vi "Course project.vi"() -> ()   [LabVIEW 2013]
uses:
  Controls/Car Race Cmd Data Cluster.ctl
  Controls/Car Race States.ctl
  Controls/Log Data Staus.ctl
  Controls/Car race Msg.ctl
  <vilib>/Utility/inputDevices.llb/keyboardAcquire.vi
panel:
  out "Speed":string
  in  "Re-Start":bool=TRUE
  out "Game Over":string
  out "Bonus":string
  out "New High Score":string
  out "Car Yellow":bool
  out "Car Race Indicator":T1
  out "User Profile":u16(ring)
  out "Message":string
  in  "Start":bool
  in  "Sign In":T2
  in  "Stop":bool
  out "Car Red":bool
  out "Race Track":u16(ring)
  # "User ID-"
  # "Password-"
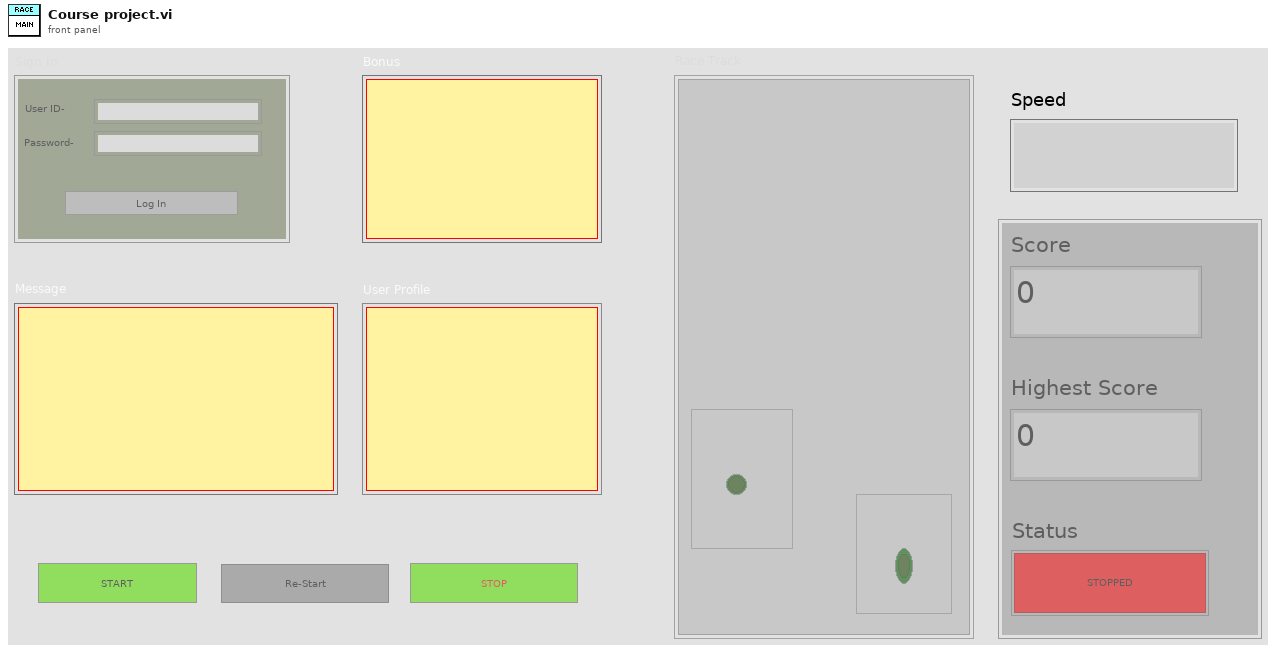
[diagram p1: front panel]
types:
  T1 = cluster{"Score":dbl, "Highest Score":dbl, "Status":bool}
  T2 = cluster{"User ID":string, "Password":string, "Log In":bool}
  T3 = typedef "Car Race Cmd Data Cluster.ctl" = cluster{"Command":T4, "Data":variant}
  T4 = typedef "Car Race States.ctl" = enum16{"Initialize", "Sign In", "Start", "Re-Start", "Game Over", "Stop"}
  T5 = cluster{"Sign In":refnum<vi>, "Race Track":refnum<vi>, "Car Red":refnum<vi>, "Car Yellow":refnum<vi>, "Car Race Indicator":refnum<vi>, "Start":refnum<vi>, "Stop":refnum<vi>, "Speed":refnum<vi>, "Re-Start":refnum<vi>}
  T6 = typedef "Car race Msg.ctl" = enum16{"Welcome Messsage", "User Inf.", "Start", "Log In Failed", "Game Over"}
  T7 = enum8{"Enabled", "Disabled", "Disabled and Grayed Out"}
  T8 = typedef "Log Data Staus.ctl" = enum16{"Initialize", "Read", "User ID Check", "Write", "Stop"}
  T9 = cluster{"First Name":string, "Last Name":string, "User ID":string, "Password":string, "Highest Score":string}
  T10 = cluster{"First Name":string, "Last Name":string, "User ID":string, "Password":string, "Highest Score":string}[]
  T11 = enum16{"0", "1", "2", "3", "4", "5", "6", "7", "8", "9", "A", "B", "C", "D", "E", "F", "G", "H", "I", "J", "K", "L", "M", "N", "O", "P", "Q", "R", "S", "T", "U", "V", "W", "X", "Y", "Z", "F1", "F2", "F3", "F4", "F5", "F6", "F7", "F8", "F9", "F10", "F11", "F12", "F13", "F14", "F15", "ADD", "BACK", "BACKSLASH", "CAPITAL", "COMMA", "DECIMAL", "DELETE", "DIVIDE", "DOWN", "END", "EQUALS", "ESCAPE", "GRAVE (`)", "HOME", "INSERT", "LBRACKET", "LCONTROL", "LEFT", "L ALT", "LSHIFT", "LWIN", "MINUS", "MULTIPLY", "NEXT", "NUMLOCK", "NUMPAD_0", "NUMPAD_1", "NUMPAD_2", "NUMPAD_3", "NUMPAD_4", "NUMPAD_5", "NUMPAD_6", "NUMPAD_7", "NUMPAD_8", "NUMPAD_9", "PAUSE", "PERIOD", "PRIOR (PG UP)", "RBRACKET", "RCONTROL", "RETURN", "RIGHT", "R ALT", "RSHIFT", "RWIN", "SCROLL", "SEMICOLON", "SLASH", "SPACE", "SUBTRACT", "TAB", "UP", "ENTER (num pad)", "' (quote)"}[]
  T12 = enum16{"0", "1", "2", "3", "4", "5", "6", "7", "8", "9", "A", "B", "C", "D", "E", "F", "G", "H", "I", "J", "K", "L", "M", "N", "O", "P", "Q", "R", "S", "T", "U", "V", "W", "X", "Y", "Z", "F1", "F2", "F3", "F4", "F5", "F6", "F7", "F8", "F9", "F10", "F11", "F12", "F13", "F14", "F15", "ADD", "BACK", "BACKSLASH", "CAPITAL", "COMMA", "DECIMAL", "DELETE", "DIVIDE", "DOWN", "END", "EQUALS", "ESCAPE", "GRAVE (`)", "HOME", "INSERT", "LBRACKET", "LCONTROL", "LEFT", "L ALT", "LSHIFT", "LWIN", "MINUS", "MULTIPLY", "NEXT", "NUMLOCK", "NUMPAD_0", "NUMPAD_1", "NUMPAD_2", "NUMPAD_3", "NUMPAD_4", "NUMPAD_5", "NUMPAD_6", "NUMPAD_7", "NUMPAD_8", "NUMPAD_9", "PAUSE", "PERIOD", "PRIOR (PG UP)", "RBRACKET", "RCONTROL", "RETURN", "RIGHT", "R ALT", "RSHIFT", "RWIN", "SCROLL", "SEMICOLON", "SLASH", "SPACE", "SUBTRACT", "TAB", "UP", "ENTER (num pad)", "' (quote)"}
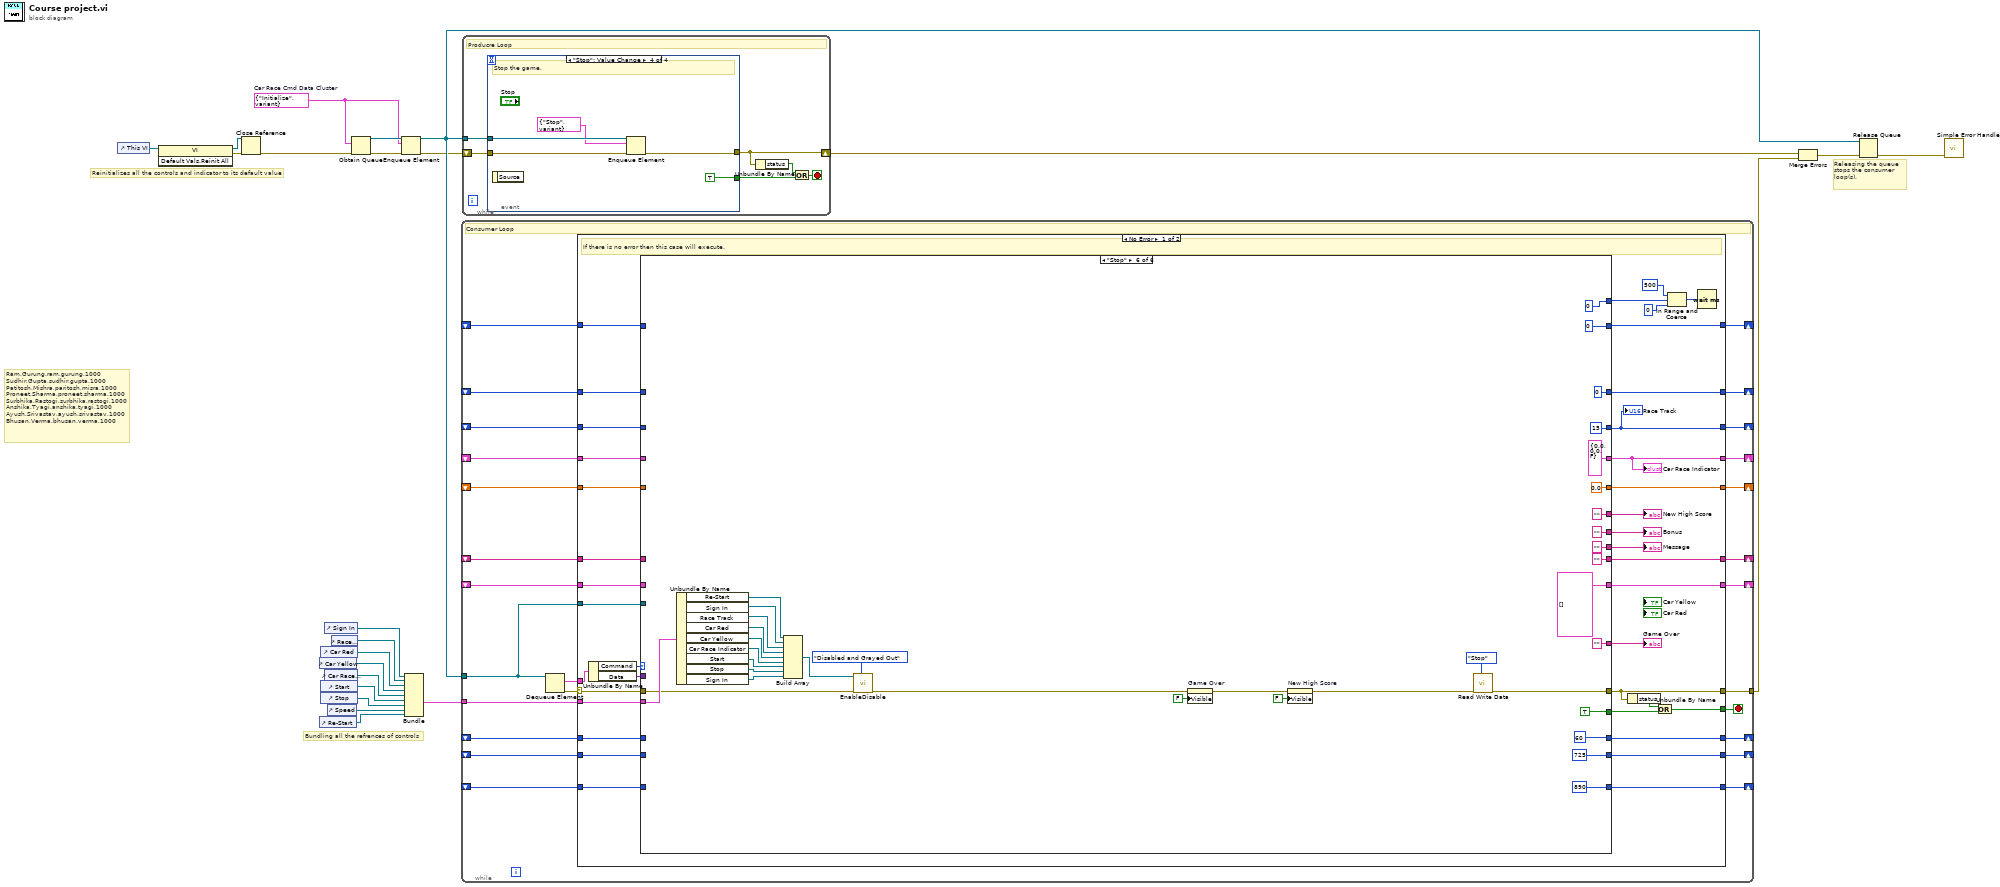
[diagram p0: block diagram]
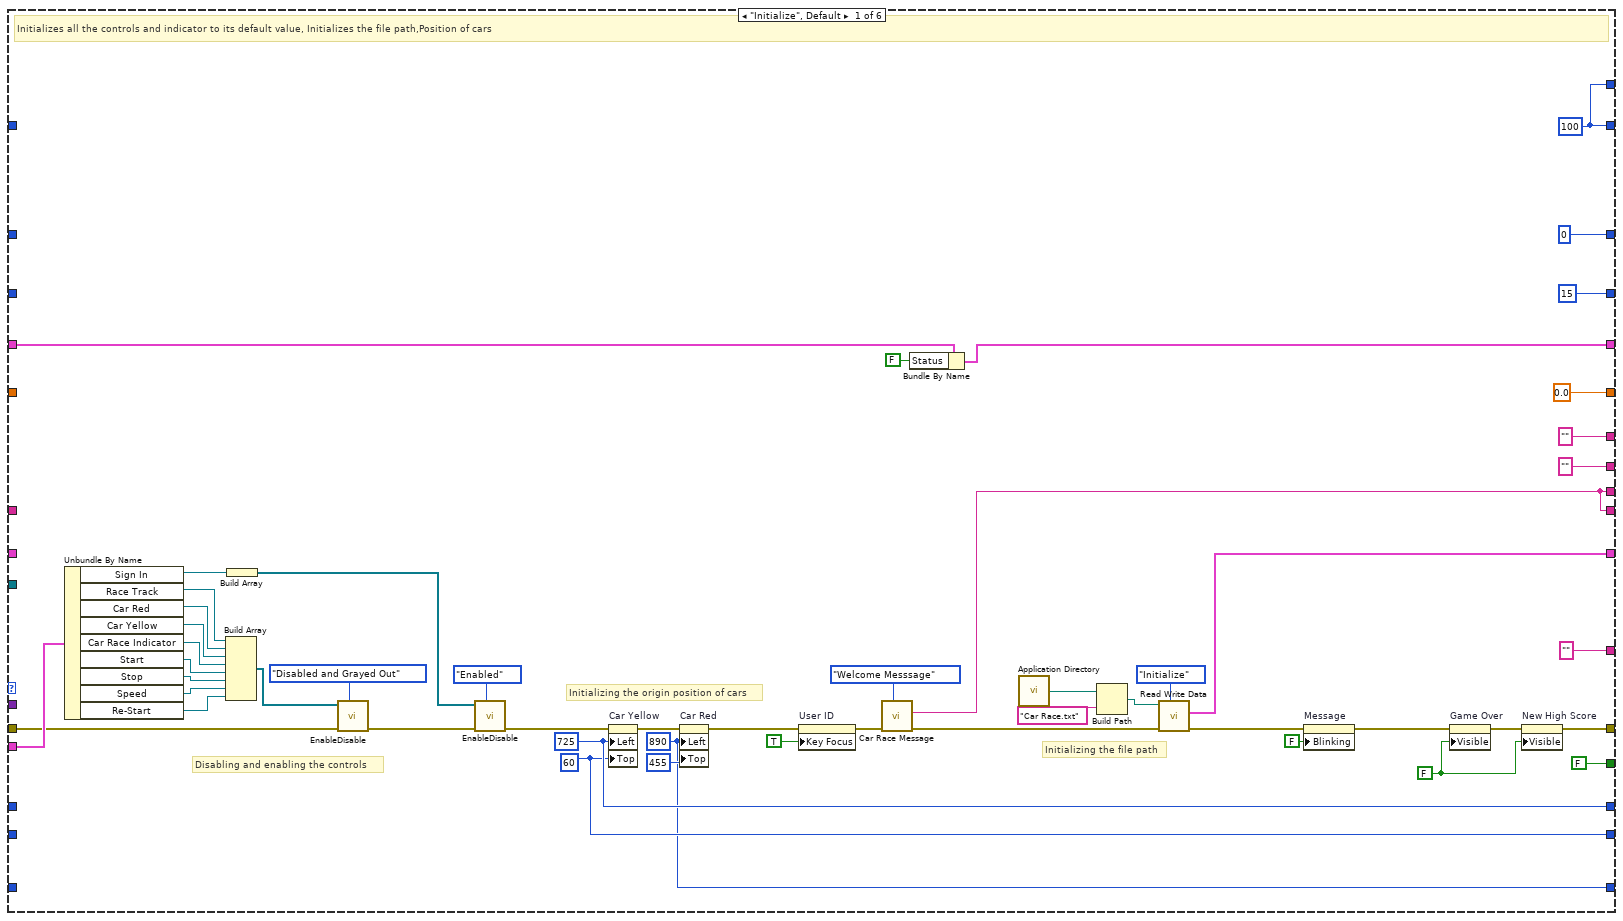
[diagram p2: hidden frame]
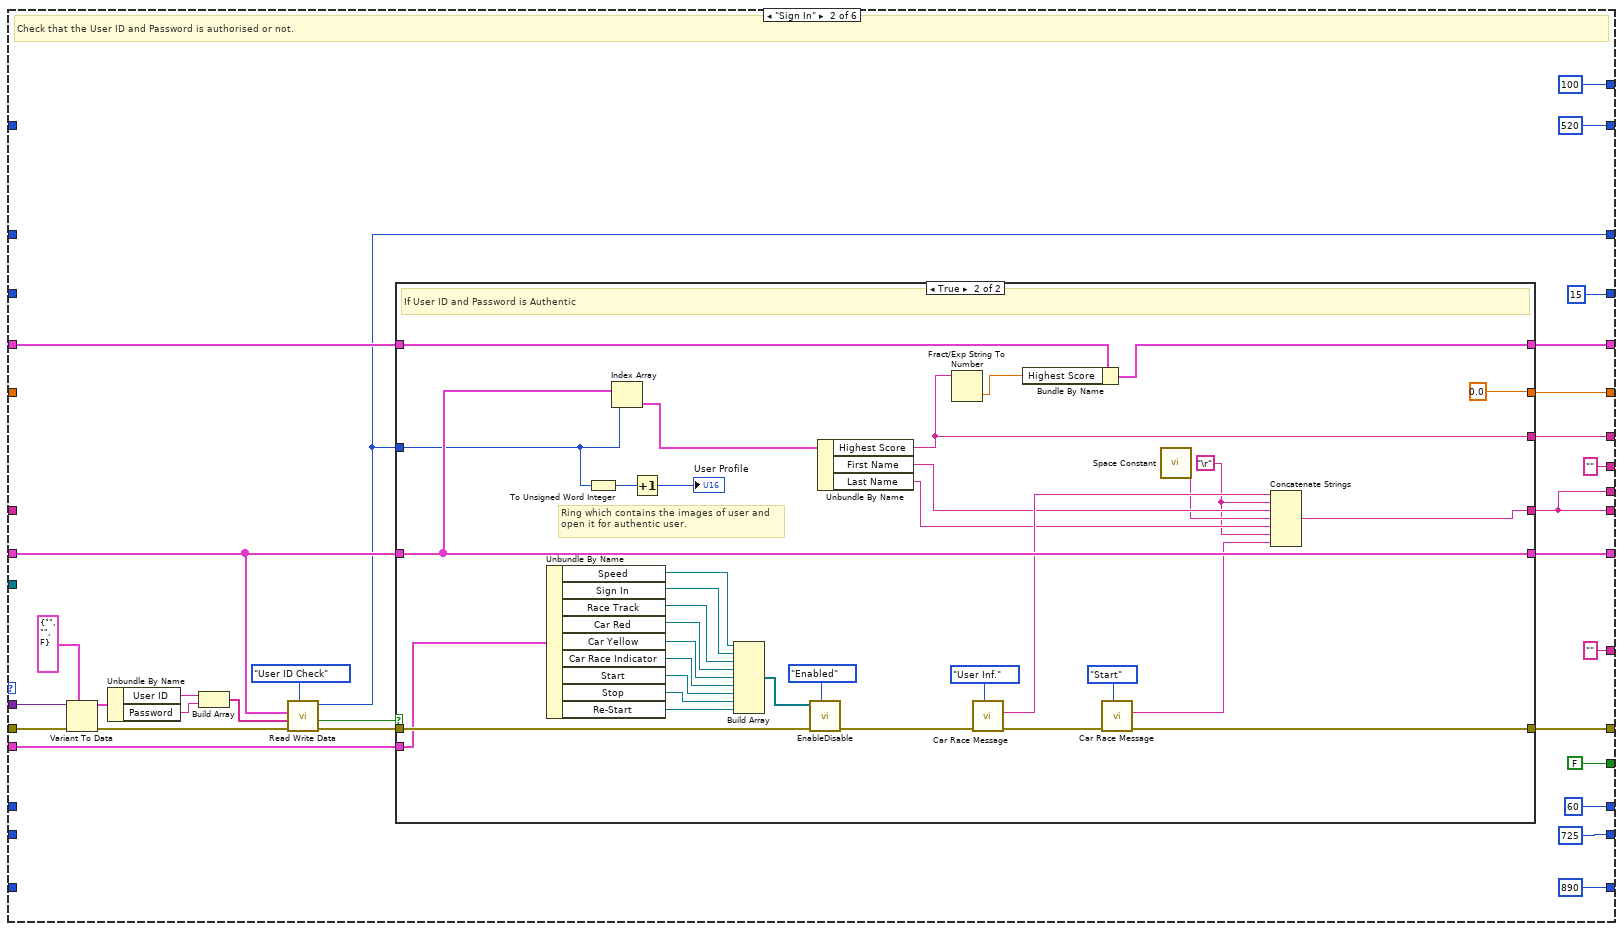
[diagram p3: hidden frame]
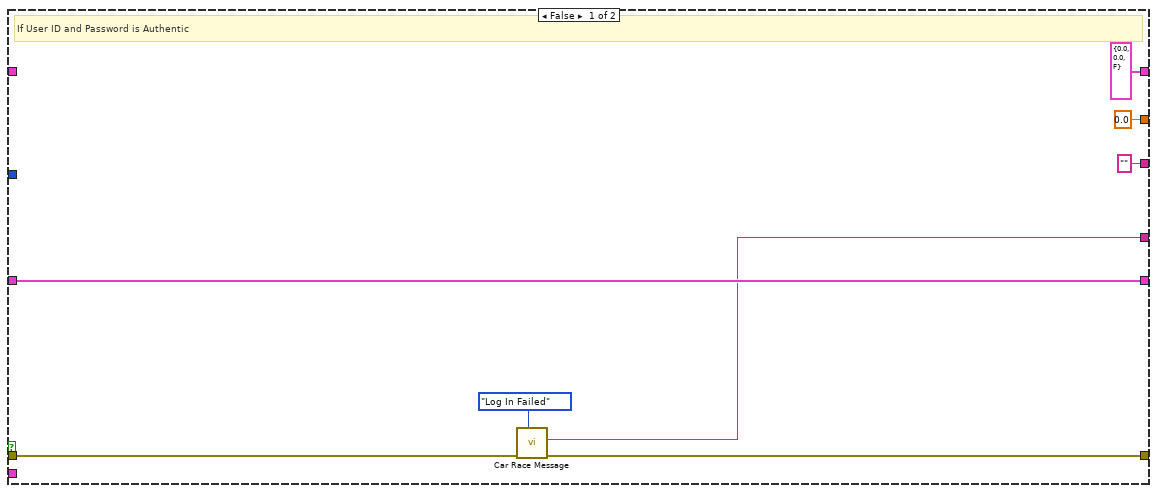
[diagram p4: hidden frame]
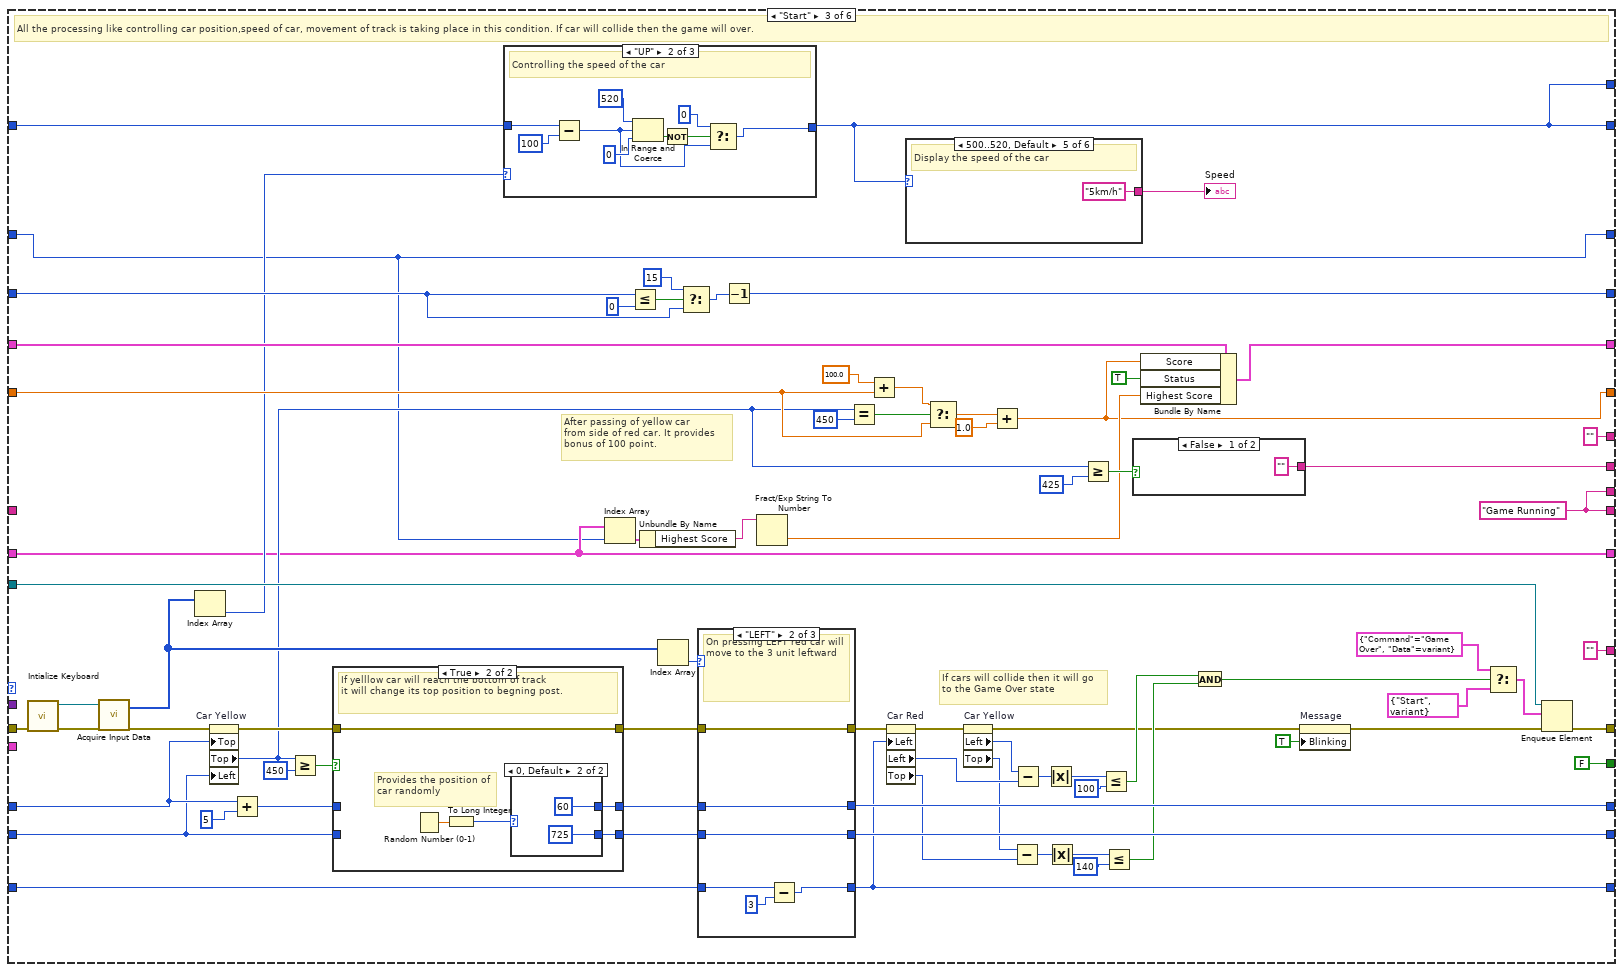
[diagram p5: hidden frame]
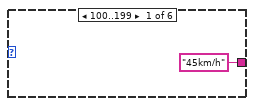
[diagram p6: hidden frame]
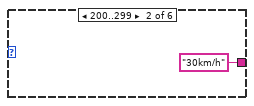
[diagram p7: hidden frame]
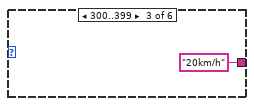
[diagram p8: hidden frame]
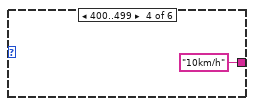
[diagram p9: hidden frame]
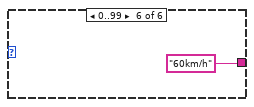
[diagram p10: hidden frame]
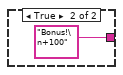
[diagram p11: hidden frame]
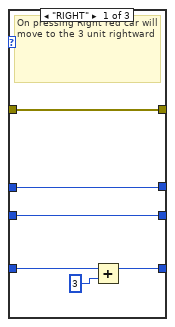
[diagram p12: hidden frame]
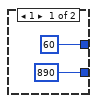
[diagram p15: hidden frame]
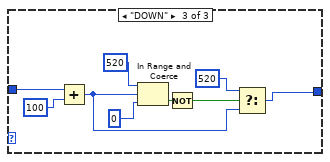
[diagram p17: hidden frame]
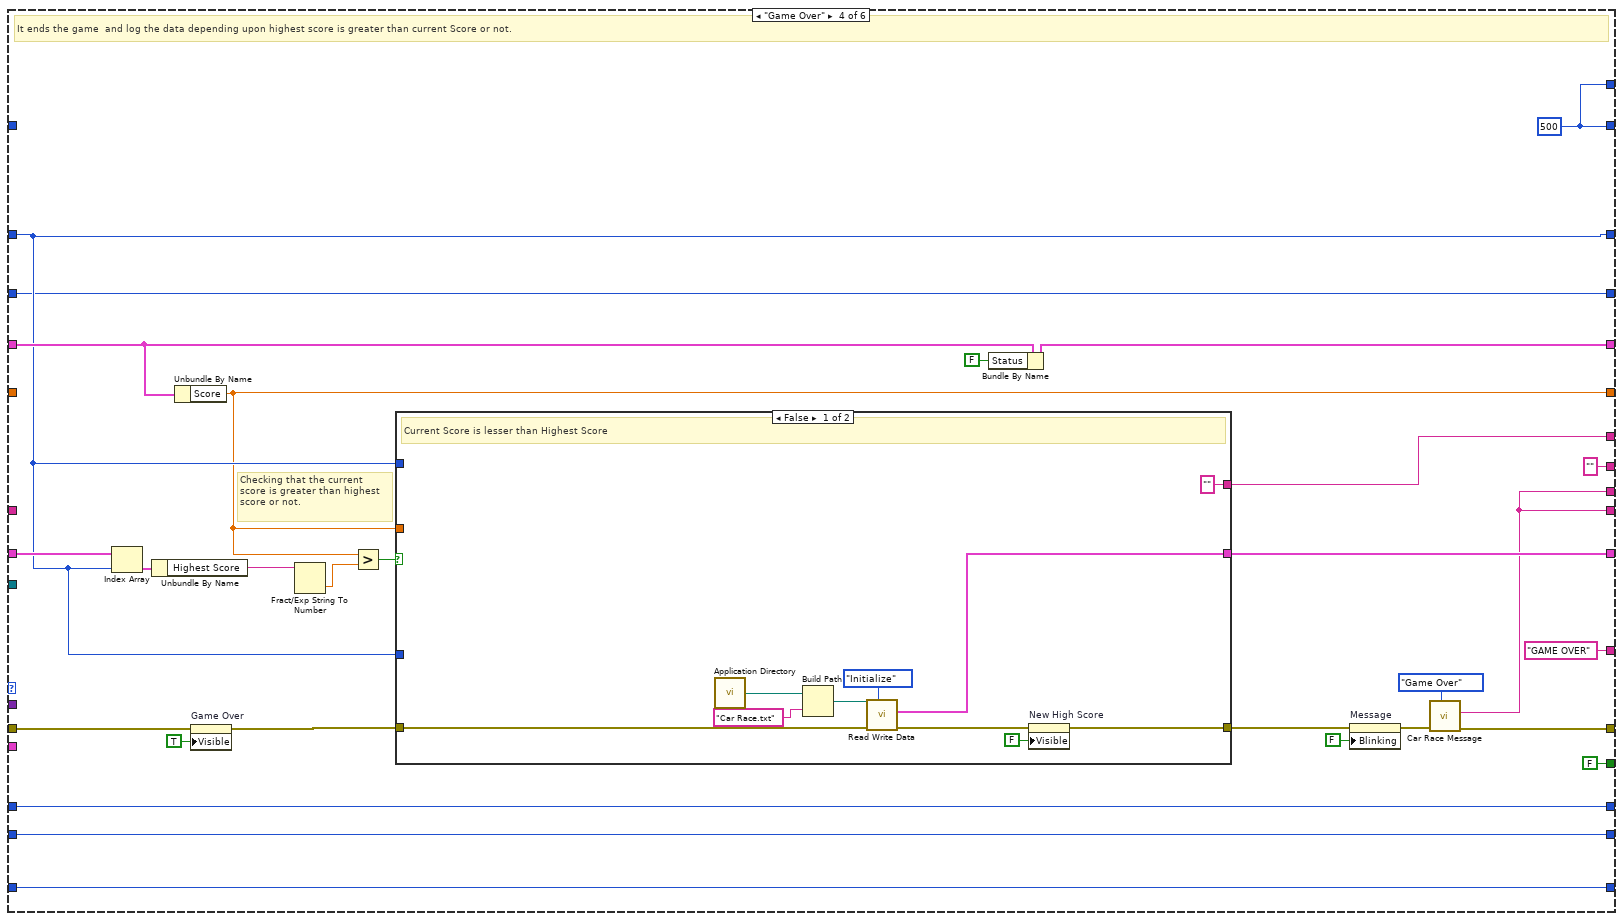
[diagram p18: hidden frame]
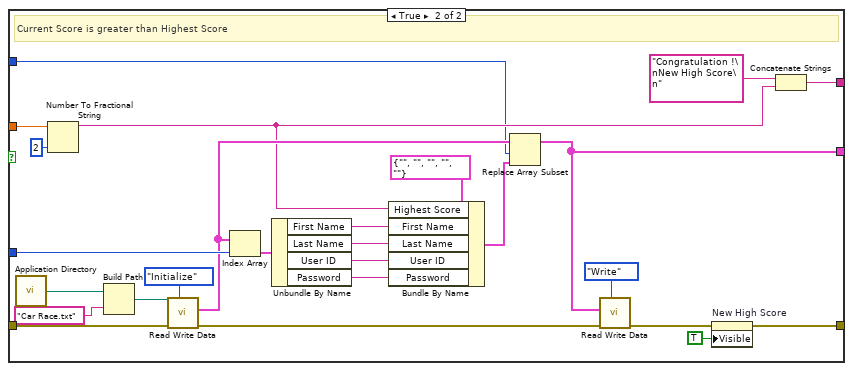
[diagram p19: hidden frame]
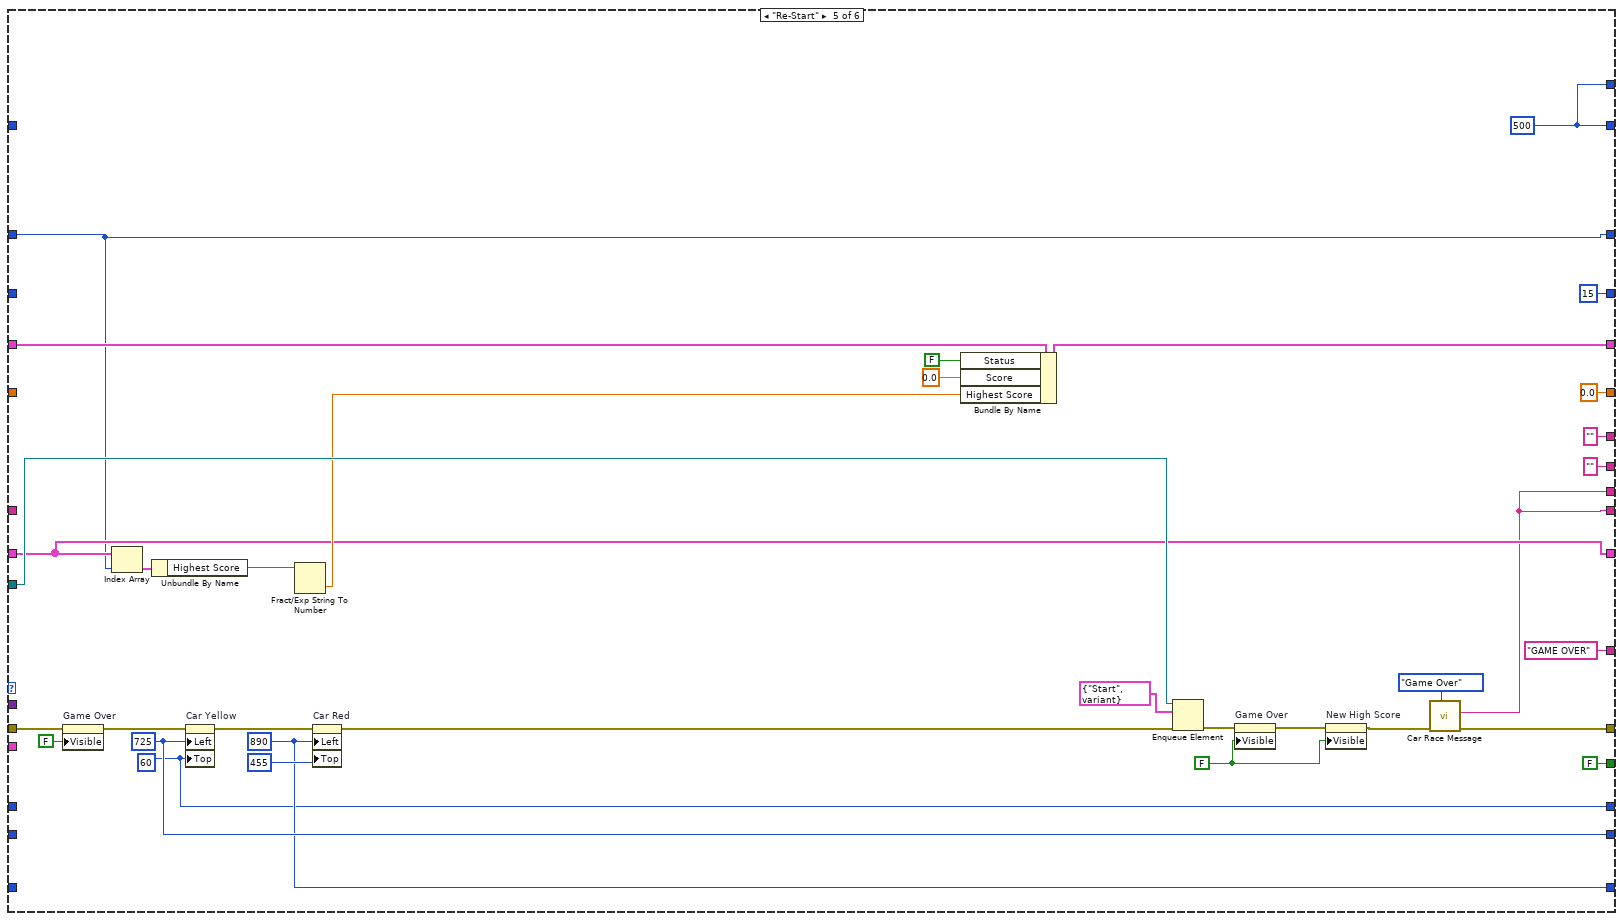
[diagram p20: hidden frame]
diagram:
  w5 = T3 {"Command"=enum."Initialize", "Data"=variant}  # Car Race Cmd Data Cluster
  # "Bundling all the refrences of controls"
  # "Releasing the queue stops the consumer loop(s)."
  # "Reinitializes all the controls and indicator to its default value"
  # "Ram,Gurung,ram,gurung,1000\nSudhir,Gupta,sudhir,gupta,1000\nPatitosh,Mishra,paritosh,misra,1000\nProneet,Sharma,proneet,sharma,1000\nSurbhika,Rastogi,surbhika,rastogi,1000\nAnshika,Tyagi,anshika,tyagi,1000\nAyush,Srivastav,ayush,srivastav,1000\nBhusan,Verma,bhusan,verma,1000"
  n1 = control-ref of="This VI"() -> (w20:refnum<vi>)
  n2 = invoke class="VI" method="Default Vals.Reinit All"(reference=w20) -> (reference out=w22:refnum<vi>, error out=w21:errorcluster)  [unwired: 2 in, 1 out]
  n3 = Close Reference(reference=w22, error in (no error)=w21) -> (error out=w16:errorcluster)
  n4 = control-ref of="Re-Start"() -> (w1:refnum<vi>)
  n5 = control-ref of="Car Yellow"() -> (w4:refnum<vi>)
  n6 = control-ref of="Car Red"() -> (w14:refnum<vi>)
  n7 = control-ref of="Start"() -> (w12:refnum<vi>)
  n8 = control-ref of="Stop"() -> (w11:refnum<vi>)
  n9 = control-ref of="Sign In"() -> (w6:refnum<vi>)
  n10 = control-ref of="Car Race Indicator"() -> (w13:refnum<vi>)
  n11 = control-ref of="Speed"() -> (w2:refnum<vi>)
  n12 = control-ref of="Race Track"() -> (w15:refnum<vi>)
  n13 = Obtain Queue(element data type=w5, error in (no error)=w16) -> (queue out=w23:refnum<queue>, error out=w18:errorcluster)  [unwired: 3 in, 1 out]
  n14 = Enqueue Element(queue=w23, element=w5, error in (no error)=w18) -> (queue out=w19:refnum<queue>, error out=w17:errorcluster)  [unwired: 1 in, 1 out]
  n15 = Bundle("Sign In"=w6, "Race Track"=w15, "Car Red"=w14, "Car Yellow"=w4, "Car Race Indicator"=w13, "Start"=w12, "Stop"=w11, "Speed"=w2, "Re-Start"=w1) -> (w10:T5)  [unwired: 1 in]
  n16 = while {
    tunnel: w19 -> [w41]
    tunnel: [w46] -> w8
    tunnel: w10 -> [w45]
    shift-right: [w44] -> _
    shift-left: _ -> [w43]
    shift-right: [w28] -> _
    shift-left: _ -> [w42]
    shift-right: [w39] -> _
    shift-left: _ -> [w40]
    shift-right: [w38] -> _
    shift-left: _ -> [w37]
    shift-right: [w36] -> _
    shift-left: _ -> [w35]
    shift-right: [w34] -> _
    shift-left: _ -> [w33]
    shift-right: [w32] -> _
    shift-left: _ -> [w31]
    shift-right: [w30] -> _
    shift-left: _ -> [w29]
    shift-right: [w27] -> _
    shift-left: _ -> [w26]
    shift-right: [w25] -> _
    shift-left: _ -> [w24]
    stop <- w47 stop-if-true
    # "Consumer Loop"
    n17 = Dequeue Element(queue=w41) -> (element=w48:T3, error out=w49:errorcluster)  [unwired: 2 in, 2 out]
    n18 = case shown="No Error" w49 {
      selector: w49 -> [w83 w488]
      tunnel: w48 -> [w80 _]
      tunnel: [w86 TRUE] -> w47
      tunnel: [w87 w488] -> w46
      tunnel: w45 -> [w82 _]
      tunnel: [w81 T10 [] ("User Information Out")] -> w44
      tunnel: w43 -> [w78 _]
      tunnel: w42 -> [w75 _]
      tunnel: [w57 T1 {"Score"=0.0, "Highest Score"=0.0, "Status"=FALSE} ("Car Race Indicator")] -> w28
      tunnel: w41 -> [w74 _]
      tunnel: w40 -> [w73 _]
      tunnel: [w72 u32 0 ("milliseconds to wait")] -> w39
      tunnel: [w65 u16 0] -> w38
      tunnel: w37 -> [w71 _]
      tunnel: [w67 "" ("Message")] -> w36
      tunnel: w35 -> [w66 _]
      tunnel: [w64 w480] -> w34
      tunnel: w33 -> [w63 w480]
      tunnel: [w62 w479] -> w32
      tunnel: w31 -> [w61 w479]
      tunnel: [w60 w478] -> w30
      tunnel: w29 -> [w59 w478]
      tunnel: [w56 0.0] -> w27
      tunnel: w26 -> [w55 _]
      tunnel: [w54 0 ("Numeric")] -> w25
      tunnel: w24 -> [w53 _]
      frame No Error {
        # "If there is no error then this case will execute."
        n19 = Unbundle By Name(w80) -> ("Command"=w79:T4, "Data"=w77:variant)
        n20 = case shown="\"Stop\"" w79 {
          tunnel: [w107 w156 w287 w357 w432 w468] -> w87
          tunnel: w83 -> [w125 w167 w285 w371 w441 w467]
          tunnel: [FALSE FALSE FALSE FALSE FALSE TRUE] -> w84
          tunnel: w82 -> [w134 w152 _ _ _ w476]
          tunnel: [w116 w154 w223 w356 w416 T10 [] ("User Information Out")] -> w81
          tunnel: w78 -> [_ w155 w223 w367 w416 _]
          tunnel: w77 -> [_ w166 _ _ _ _]
          tunnel: [w98 w146 w218 w354 w414 "" ("Message")] -> w76
          tunnel: w75 -> [w105 w151 w273 w368 w438 _]
          tunnel: [w104 w150 w240 w361 w435 T1 {"Score"=0.0, "Highest Score"=0.0, "Status"=FALSE} ("Car Race Indicator")] -> w57
          tunnel: w74 -> [_ _ w286 _ w423 _]
          tunnel: w73 -> [_ _ w282 _ _ _]
          tunnel: [w94 u32 520 w225 w343 w408 u32 0 ("lower limit")] -> w72
          tunnel: [u16 15 u16 15 w280 w350 u16 15 u16 15] -> w65
          tunnel: w71 -> [_ _ w278 w350 _ _]
          tunnel: [w94 u32 100 ("y") w225 w343 w408 u32 0 ("y")] -> w68
          tunnel: [w98 w146 w218 w354 w414 "" ("Message")] -> w67
          tunnel: w66 -> [_ _ _ _ _ _]
          tunnel: [w97 60 w263 w347 w424 60 ("Position:Top")] -> w64
          tunnel: w63 -> [_ _ w272 w347 _ _]
          tunnel: [w96 725 w261 w346 w426 725 ("Position:Left")] -> w62
          tunnel: w61 -> [_ _ w268 w346 _ _]
          tunnel: [w95 890 w252 w345 w425 890 ("Position:Left")] -> w60
          tunnel: w59 -> [_ _ w267 w345 _ _]
          tunnel: ["" "" "" "GAME OVER" "GAME OVER" ""] -> w58
          tunnel: [0.0 w142 w211 w349 0.0 ("Score") 0.0 ("Score")] -> w56
          tunnel: w55 -> [_ _ w236 _ _ _]
          tunnel: [0 ("Numeric") w141 w222 w355 w415 0 ("Numeric")] -> w54
          tunnel: w53 -> [_ _ w222 w355 w415 _]
          tunnel: ["" w140 "" ("Highest Score") w362 "" ("Highest Score") "" ("Highest Score")] -> w52
          tunnel: ["" "" w230 "" "" ""] -> w51
          frame "Initialize", Default {
            w106 = FALSE ("Visible")
            w94 = u32 100 ("y")
            w95 = 890 ("Position:Left")
            w97 = 725 ("Position:Left")
            w96 = 60 ("Position:Top")
            # "Initializing the file path"
            # "Initializing the origin position of cars"
            # "Disabling and enabling the controls"
            # "Initializes all the controls and indicator to its default value, Initializes the file path,Position of cars"
            n21 = Unbundle By Name(w134) -> ("Sign In"=w126:refnum<vi>, "Race Track"=w133:refnum<vi>, "Car Red"=w132:refnum<vi>, "Car Yellow"=w131:refnum<vi>, "Car Race Indicator"=w130:refnum<vi>, "Start"=w129:refnum<vi>, "Stop"=w128:refnum<vi>, "Speed"=w127:refnum<vi>, "Re-Start"=w102:refnum<vi>)
            n22 = Build Array(w133, w132, w131, w130, w129, w128, w127, w102) -> (w124:refnum<vi>[])
            n23 = Build Array(w126) -> (w120:refnum<vi>[])
            n24 = call "EnableDisable.vi"("Command"=T7."Disabled and Grayed Out" ("Disabled"), "error in"=w125, "Array"=w124) -> ("error out"=w122:errorcluster)  [unwired: 8 in]
            n25 = call "EnableDisable.vi"("Command"=T7."Enabled", "error in"=w122, "Array"=w120) -> ("error out"=w110:errorcluster)  [unwired: 8 in]
            n26 = property on="Car Yellow" class="Bool (strict)"(error in=w110, "Left"=w97, "Top"=w96) -> (error out=w109:errorcluster)  [unwired: 1 in, 1 out]
            n27 = property on="Car Red" class="Bool (strict)"(error in=w109, "Left"=w95, "Top"=455 ("Position:Top")) -> (error out=w111:errorcluster)  [unwired: 1 in, 1 out]
            n28 = property on="User ID" class="Str"(error in=w111, "Key Focus"=TRUE) -> (error out=w115:errorcluster)  [unwired: 1 in, 1 out]
            n29 = call "Car Race Message.vi"(7:Car_race_Msg."Welcome Messsage", "error in"=w115) -> ("error IO"=w114:errorcluster, "Message"=w98:string)  [unwired: 8 in]
            n30 = Bundle By Name(cluster=w105, "Status"=FALSE) -> (w104:T1)
            n31 = call <vilib>:"Application Directory.vi"() -> ("Application Directory"=w119:path)
            n32 = Build Path(base path=w119, name or relative path="Car Race.txt") -> (appended path=w117:path)
            n33 = call "Read Write Data.vi"("Enum"=Log_Data_Staus."Initialize", "error in (no error)"=w114, "file path"=w117) -> ("error out"=w101:errorcluster, "User Information Out"=w116:T10)  [unwired: 5 in, 2 out]
            n34 = property on="Message" class="Str"(error in=w101, "Blinking"=FALSE ("Visible")) -> (error out=w100:errorcluster)  [unwired: 1 in, 1 out]
            n35 = property on="Game Over" class="Str"(error in=w100, "Visible"=w106) -> (error out=w108:errorcluster)  [unwired: 1 in, 1 out]
            n36 = property on="New High Score" class="Str"(error in=w108, "Visible"=w106) -> (error out=w107:errorcluster)  [unwired: 1 in, 1 out]
          }
          frame "Sign In" {
            # "Check that the User ID and Password is authorised or not."
            n37 = Variant To Data(error in=w167, type=T2 {"User ID"="", "Password"="", "Log In"=FALSE} ("Sign In"), Variant=w166) -> (data=w164:T2, error out=w163:errorcluster)
            n38 = Unbundle By Name(w164) -> ("User ID"=w162:string, "Password"=w161:string)
            n39 = Build Array(w162, w161) -> (w160:string[])
            n40 = call "Read Write Data.vi"("Enum"=Log_Data_Staus."User ID Check", "error in (no error)"=w163, "Sign In Detail"=w160, "User Information In"=w155) -> ("error out"=w157:errorcluster, "Boolean"=w153:bool, "Numeric"=w141:i32)  [unwired: 4 in, 1 out]
            n41 = case shown="True" w153 {
              tunnel: w157 -> [w174 w200]
              tunnel: [w173 w179] -> w156
              tunnel: w155 -> [w175 w196]
              tunnel: [w175 w196] -> w154
              tunnel: w152 -> [_ w199]
              tunnel: [w171 w187] -> w146
              tunnel: [T1 {"Score"=0.0, "Highest Score"=0.0, "Status"=FALSE} ("Car Race Indicator") w194] -> w150
              tunnel: w151 -> [_ w197]
              tunnel: w141 -> [_ w192]
              tunnel: [0.0 0.0] -> w142
              tunnel: ["" ("Highest Score") w176] -> w140
              frame False {
                # "If User ID and Password is Authentic"
                n42 = call "Car Race Message.vi"(7:Car_race_Msg."Log In Failed", "error in"=w174) -> ("error IO"=w173:errorcluster, "Message"=w171:string)  [unwired: 8 in]
              }
              frame True {
                w178 = "\r"
                # "Ring which contains the images of user and open it for authentic user."
                # "If User ID and Password is Authentic"
                n43 = Unbundle By Name(w199) -> ("Speed"=w182:refnum<vi>, "Sign In"=w201:refnum<vi>, "Race Track"=w210:refnum<vi>, "Car Red"=w209:refnum<vi>, "Car Yellow"=w208:refnum<vi>, "Car Race Indicator"=w207:refnum<vi>, "Start"=w206:refnum<vi>, "Stop"=w205:refnum<vi>, "Re-Start"=w204:refnum<vi>)
                n44 = To Unsigned Word Integer(number=w192) -> (unsigned 16bit integer=w191:u16)
                n45 = Index Array(array=w196, index=w192) -> (element=w195:T9)
                n46 = Increment(x=w191) -> (x+1=→"User Profile":u16)
                n47 = Build Array(w182, w201, w210, w209, w208, w207, w206, w205, w204) -> (w203:refnum<vi>[])
                n48 = call "EnableDisable.vi"("Command"=T7."Enabled" ("Disabled"), "error in"=w200, "Array"=w203) -> ("error out"=w198:errorcluster)  [unwired: 8 in]
                n49 = Unbundle By Name(w195) -> ("Highest Score"=w176:string, "First Name"=w185:string, "Last Name"=w183:string)
                n50 = Fract/Exp String To Number(string=w176) -> (number=w193:dbl)  [unwired: 3 in, 1 out]
                n51 = call "Car Race Message.vi"(7:Car_race_Msg."User Inf.", "error in"=w198) -> ("error IO"=w180:errorcluster, "Message"=w186:string)  [unwired: 8 in]
                n52 = Bundle By Name(cluster=w197, "Highest Score"=w193) -> (w194:T1)
                n53 = call "Car Race Message.vi"(7:Car_race_Msg."Start", "error in"=w180) -> ("error IO"=w179:errorcluster, "Message"=w177:string)  [unwired: 8 in]
                n54 = call <vilib>:"Space Constant.vi"() -> ("String"=w184:string)
                n55 = Concatenate Strings(w186, w178, w185, w184, w183, w178, w177) -> (w187:string)
              }
            }
          }
          frame "Start" {
            w218 = "Game Running"
            # "If cars will collide then it will go to the Game Over state"
            # "After passing of yellow car \nfrom side of red car. It provides \nbonus of 100 point."
            # "All the processing like controlling car position,speed of car, movement of track is taking place in this condition. If car will collide then the game will over."
            n56 = call <vilib>:"Intialize Keyboard.vi"("error in (no error)"=w285) -> ("error out"=w284:errorcluster, "device ID"=w283:refnum<k1>)  [unwired: 9 in]
            n57 = call-poly <vilib>:"Acquire Input Data.vi"("device ID"=w283, "error in (no error)"=w284) -> ("keys pressed"=w266:T11, "error out"=w275:errorcluster)  [unwired: 15 in, 1 out]
            n58 = Index Array(array=w266) -> (element=w226:T12)  [unwired: 1 in]
            n59 = property on="Car Yellow" class="Bool (strict)"(error in=w275, "Top"=w272, "Left"=w268) -> (error out=w270:errorcluster, "Top"=w229:i32)  [unwired: 1 in, 1 out]
            n60 = Add(x=w272, y=5) -> (x+y=w269:i32)
            n61 = Greater Or Equal?(x=w229, y=450) -> (x >= y?=w231:bool)
            n62 = case shown="True" w231 {
              tunnel: w270 -> [w314 w319]
              tunnel: [w314 w319] -> w259
              tunnel: w269 -> [w313 _]
              tunnel: [w313 w318] -> w264
              tunnel: w268 -> [w312 _]
              tunnel: [w312 w317] -> w262
              frame False {
              }
              frame True {
                # "Provides the position of car randomly"
                # "If yelllow car will reach the bottom of track \nit will change its top position to begning post."
                n63 = Random Number (0-1)() -> (number: 0 to 1=w316:dbl)
                n64 = To Long Integer(number=w316) -> (32bit integer=w315:i32)
                n65 = case shown="0, Default" w315 {
                  tunnel: [60 60] -> w318
                  tunnel: [890 725] -> w317
                  frame 1 {
                  }
                  frame 0, Default {
                  }
                }
              }
            }
            n66 = case shown="\"UP\"" w226 {
              tunnel: [w324 w326 w335] -> w225
              tunnel: w282 -> [w324 w332 w341]
              frame "0", Default {
              }
              frame "UP" {
                # "Controlling the speed of the car"
                n67 = Subtract(x=w332, y=u32 100) -> (x-y=w327:u32)
                n68 = In Range and Coerce(upper limit=u32 520, x=w327, lower limit=u32 0) -> (In Range?=w329:bool)  [unwired: 1 out]
                n69 = Not(x=w329) -> (.not. x?=w325:bool)
                n70 = Select(t=u32 0 ("lower limit"), s=w325, f=w327) -> (s? t:f=w326:u32)
              }
              frame "DOWN" {
                n71 = Add(x=w341, y=u32 100) -> (x+y=w336:u32)
                n72 = In Range and Coerce(upper limit=u32 520, x=w336, lower limit=u32 0) -> (In Range?=w338:bool)  [unwired: 1 out]
                n73 = Not(x=w338) -> (.not. x?=w334:bool)
                n74 = Select(t=u32 520 ("lower limit"), s=w334, f=w336) -> (s? t:f=w335:u32)
              }
            }
            n75 = Index Array(array=w223, index=w222) -> (element=w221:T9)
            n76 = Less Or Equal?(x=w278, y=u16 0) -> (x <= y?=w281:bool)
            n77 = Unbundle By Name(w221) -> ("Highest Score"=w220:string)
            n78 = Index Array(array=w266) -> (element=w265:T12)  [unwired: 1 in]
            n79 = Select(t=u16 15, s=w281, f=w278) -> (s? t:f=w279:u16)
            n80 = case shown="\"LEFT\"" w265 {
              tunnel: [w298 w306 w311] -> w252
              tunnel: w267 -> [w301 w307 w311]
              tunnel: [w299 w304 w310] -> w263
              tunnel: w264 -> [w299 w304 w310]
              tunnel: w262 -> [w300 w303 w309]
              tunnel: [w300 w303 w309] -> w261
              tunnel: [w296 w302 w308] -> w260
              tunnel: w259 -> [w296 w302 w308]
              frame "RIGHT" {
                # "On pressing Right red car will move to the 3 unit rightward"
                n81 = Add(x=w301, y=3) -> (x+y=w298:i32)
              }
              frame "LEFT" {
                # "On pressing LEFT red car will move to the 3 unit leftward"
                n82 = Subtract(x=w307, y=3 ("x")) -> (x-y=w306:i32)
              }
              frame "UP", Default {
              }
            }
            n83 = Decrement(x=w279) -> (x-1=w280:u16)
            n84 = Fract/Exp String To Number(string=w220) -> (number=w219:dbl)  [unwired: 3 in, 1 out]
            n85 = Equal?(x=w229, y=450) -> (x = y?=w232:bool)
            n86 = Add(x=100.0, y=w236) -> (x+y=w237:dbl)
            n87 = property on="Car Red" class="Bool (strict)"(error in=w260, "Left"=w252) -> (error out=w258:errorcluster, "Left"=w256:i32, "Top"=w247:i32)  [unwired: 1 in, 1 out]
            n88 = case shown="500..520, Default" w225 {
              tunnel: ["45km/h" "30km/h" "20km/h" "10km/h" "5km/h" "60km/h"] -> w224
              frame 100..199 {
              }
              frame 200..299 {
              }
              frame 300..399 {
              }
              frame 400..499 {
              }
              frame 500..520, Default {
                # "Display the speed of the car"
              }
              frame 0..99 {
              }
            }
            "Speed" <- w224
            n89 = Select(t=w237, s=w232, f=w236) -> (s? t:f=w234:dbl)
            n90 = property on="Car Yellow" class="Bool (strict)"(error in=w258) -> (error out=w217:errorcluster, "Left"=w257:i32, "Top"=w253:i32)  [unwired: 1 in, 1 out]
            n91 = Add(x=w234, y=1.0) -> (x+y=w211:dbl)
            n92 = Subtract(x=w253, y=w247) -> (x-y=w250:i32)
            n93 = Subtract(x=w257, y=w256) -> (x-y=w255:i32)
            n94 = Absolute Value(x=w255) -> (abs(x)=w251:i32)
            n95 = Absolute Value(x=w250) -> (abs(x)=w249:i32)
            n96 = Greater Or Equal?(x=w229, y=425) -> (x >= y?=w227:bool)
            n97 = Less Or Equal?(x=w251, y=100) -> (x <= y?=w246:bool)
            n98 = Less Or Equal?(x=w249, y=140) -> (x <= y?=w245:bool)
            n99 = case shown="False" w227 {
              tunnel: ["" "Bonus!\n+100"] -> w230
              frame False {
              }
              frame True {
              }
            }
            n100 = Bundle By Name(cluster=w273, "Score"=w211, "Status"=TRUE, "Highest Score"=w219) -> (w240:T1)
            n101 = And(x=w246, y=w245) -> (x .and. y?=w244:bool)
            n102 = property on="Message" class="Str"(error in=w217, "Blinking"=TRUE) -> (error out=w216:errorcluster)  [unwired: 1 in, 1 out]
            n103 = Select(t=T3 {"Command"=enum."Game Over", "Data"=variant} ("element"), s=w244, f=T3 {"Command"=enum."Start", "Data"=variant}) -> (s? t:f=w241:T3)
            n104 = Enqueue Element(queue=w286, element=w241, error in (no error)=w216) -> (error out=w287:errorcluster)  [unwired: 1 in, 2 out]
          }
          frame "Game Over" {
            w343 = u32 500 ("upper limit")
            # "Checking that the current score is greater than highest score or not."
            # "It ends the game  and log the data depending upon highest score is greater than current Score or not."
            n105 = Index Array(array=w367, index=w355) -> (element=w366:T9)
            n106 = Unbundle By Name(w366) -> ("Highest Score"=w365:string)
            n107 = Unbundle By Name(w368) -> ("Score"=w349:dbl)
            n108 = property on="Game Over" class="Str"(error in=w371, "Visible"=TRUE) -> (error out=w359:errorcluster)  [unwired: 1 in, 1 out]
            n109 = Fract/Exp String To Number(string=w365) -> (number=w364:dbl)  [unwired: 3 in, 1 out]
            n110 = Greater?(x=w349, y=w364) -> (0:w363:bool)
            n111 = case shown="False" w363 {
              tunnel: w359 -> [w374 w406]
              tunnel: [w380 w392] -> w352
              tunnel: w355 -> [_ w402]
              tunnel: w349 -> [_ w396]
              tunnel: ["" w390] -> w362
              tunnel: w355 -> [_ w386]
              tunnel: [w372 w382] -> w356
              frame False {
                # "Current Score is lesser than Highest Score"
                n112 = call <vilib>:"Application Directory.vi"() -> ("Application Directory"=w377:path)
                n113 = Build Path(base path=w377, name or relative path="Car Race.txt") -> (appended path=w375:path)
                n114 = call "Read Write Data.vi"("Enum"=Log_Data_Staus."Initialize", "error in (no error)"=w374, "file path"=w375) -> ("error out"=w373:errorcluster, "User Information Out"=w372:T10)  [unwired: 5 in, 2 out]
                n115 = property on="New High Score" class="Str"(error in=w373, "Visible"=FALSE) -> (error out=w380:errorcluster)  [unwired: 1 in, 1 out]
              }
              frame True {
                # "Current Score is greater than Highest Score"
                n116 = call <vilib>:"Application Directory.vi"() -> ("Application Directory"=w385:path)
                n117 = Number To Fractional String(number=w396, precision (6)=i16 2) -> (F-format string=w388:string)  [unwired: 2 in]
                n118 = Build Path(base path=w385, name or relative path="Car Race.txt") -> (appended path=w383:path)
                n119 = call "Read Write Data.vi"("Enum"=Log_Data_Staus."Initialize", "error in (no error)"=w406, "file path"=w383) -> ("error out"=w405:errorcluster, "User Information Out"=w395:T10)  [unwired: 5 in, 2 out]
                n120 = Index Array(array=w395, index=w402) -> (element=w403:T9)
                n121 = Unbundle By Name(w403) -> ("First Name"=w400:string, "Last Name"=w399:string, "User ID"=w398:string, "Password"=w397:string)
                n122 = Bundle By Name(cluster=T9 {"First Name"="", "Last Name"="", "User ID"="", "Password"="", "Highest Score"=""}, "Highest Score"=w388, "First Name"=w400, "Last Name"=w399, "User ID"=w398, "Password"=w397) -> (w394:T9)
                n123 = Replace Array Subset(array=w395, new element=w394, index=w386) -> (w382:T10)
                n124 = call "Read Write Data.vi"("Enum"=Log_Data_Staus."Write", "error in (no error)"=w405, "User Information In"=w382) -> ("error out"=w393:errorcluster)  [unwired: 5 in, 3 out]
                n125 = property on="New High Score" class="Str"(error in=w393, "Visible"=TRUE) -> (error out=w392:errorcluster)  [unwired: 1 in, 1 out]
                n126 = Concatenate Strings("Congratulation !\nNew High Score\n", w388) -> (w390:string)
              }
            }
            n127 = Bundle By Name(cluster=w368, "Status"=FALSE) -> (w361:T1)
            n128 = property on="Message" class="Str"(error in=w352, "Blinking"=FALSE) -> (error out=w351:errorcluster)  [unwired: 1 in, 1 out]
            n129 = call "Car Race Message.vi"(7:Car_race_Msg."Game Over", "error in"=w351) -> ("error IO"=w357:errorcluster, "Message"=w354:string)  [unwired: 8 in]
          }
          frame "Re-Start" {
            w408 = u32 500 ("upper limit")
            w419 = FALSE ("Visible")
            w425 = 890 ("Position:Left")
            w426 = 725 ("Position:Left")
            w424 = 60 ("Position:Top")
            n130 = property on="Game Over" class="Str"(error in=w441, "Visible"=FALSE) -> (error out=w428:errorcluster)  [unwired: 1 in, 1 out]
            n131 = Index Array(array=w416, index=w415) -> (element=w437:T9)
            n132 = Unbundle By Name(w437) -> ("Highest Score"=w436:string)
            n133 = property on="Car Yellow" class="Bool (strict)"(error in=w428, "Left"=w426, "Top"=w424) -> (error out=w430:errorcluster)  [unwired: 1 in, 1 out]
            n134 = Fract/Exp String To Number(string=w436) -> (number=w417:dbl)  [unwired: 3 in, 1 out]
            n135 = property on="Car Red" class="Bool (strict)"(error in=w430, "Left"=w425, "Top"=455 ("Position:Top")) -> (error out=w427:errorcluster)  [unwired: 1 in, 1 out]
            n136 = Bundle By Name(cluster=w438, "Status"=FALSE, "Score"=0.0, "Highest Score"=w417) -> (w435:T1)
            n137 = Enqueue Element(queue=w423, element=T3 {"Command"=enum."Start", "Data"=variant}, error in (no error)=w427) -> (error out=w421:errorcluster)  [unwired: 1 in, 2 out]
            n138 = property on="Game Over" class="Str"(error in=w421, "Visible"=w419) -> (error out=w422:errorcluster)  [unwired: 1 in, 1 out]
            n139 = property on="New High Score" class="Str"(error in=w422, "Visible"=w419) -> (error out=w420:errorcluster)  [unwired: 1 in, 1 out]
            n140 = call "Car Race Message.vi"(7:Car_race_Msg."Game Over", "error in"=w420) -> ("error IO"=w432:errorcluster, "Message"=w414:string)  [unwired: 8 in]
          }
          frame "Stop" {
            n141 = Unbundle By Name(w476) -> ("Re-Start"=w442:refnum<vi>, "Sign In"=w464:refnum<vi>, "Race Track"=w475:refnum<vi>, "Car Red"=w474:refnum<vi>, "Car Yellow"=w473:refnum<vi>, "Car Race Indicator"=w472:refnum<vi>, "Start"=w471:refnum<vi>, "Stop"=w470:refnum<vi>, "Sign In"=w469:refnum<vi>)
            n142 = Build Array(w442, w464, w475, w474, w473, w472, w471, w470, w469) -> (w466:refnum<vi>[])
            n143 = call "EnableDisable.vi"("Command"=T7."Disabled and Grayed Out" ("Disabled"), "error in"=w467, "Array"=w466) -> ("error out"=w459:errorcluster)  [unwired: 8 in]
            n144 = property on="Game Over" class="Str"(error in=w459, "Visible"=FALSE) -> (error out=w458:errorcluster)  [unwired: 1 in, 1 out]
            n145 = property on="New High Score" class="Str"(error in=w458, "Visible"=FALSE) -> (error out=w457:errorcluster)  [unwired: 1 in, 1 out]
            n146 = call "Read Write Data.vi"("Enum"=Log_Data_Staus."Stop", "error in (no error)"=w457) -> ("error out"=w468:errorcluster)  [unwired: 6 in, 3 out]
          }
        }
        "Message" <- w76
        "Car Race Indicator" <- w57
        "Race Track" <- w65
        "Game Over" <- w58
        "New High Score" <- w52
        "Bonus" <- w51
        n147 = Unbundle By Name(w87) -> ("status"=w85:bool)
        n148 = Or(x=w85, y=w84) -> (x .or. y?=w86:bool)
        n149 = In Range and Coerce(upper limit=u32 500, x=w68, lower limit=u32 0) -> (coerced(x)=w69:u32)  [unwired: 1 out]
        n150 = Wait (ms)(milliseconds to wait=w69) -> ()  [unwired: 1 out]
      }
      frame Error {
        # "If there is error then this case will execute."
      }
    }
  }
  n151 = while {
    shift-right: [w491] -> w3
    shift-left: w17 -> [w494]
    tunnel: w19 -> [w495]
    stop <- w492 stop-if-true
    # "Producre Loop"
    n152 = event shown="[3] \"Stop\": Value Change" {
      selector: _ -> [_ _ _ _]
      dyn-events: _ -> [_ _ _ _]
      timeout: _ -> [_ _ _ _]
      tunnel: w495 -> [w501 w506 w514 w518]
      tunnel: w494 -> [w503 w508 w510 w520]
      tunnel: [w502 w507 w515 w519] -> w491
      tunnel: [FALSE ("Stop") FALSE ("Stop") FALSE ("Stop") TRUE ("Stop")] -> w493
      event "Sign In.Log In": Value Change {
        # "Transfer the data provided by the user to sign In. And go to Sign In case"
        n153 = event-data() -> ()  [unwired: 1 in, 1 out]
        n154 = To Variant(anything="Sign In") -> (Variant=w497:variant)
        n155 = Bundle By Name(cluster=T3 {"Command"=enum."Sign In", "Data"=variant} ("Car Race Cmd Data Cluster"), "Data"=w497) -> (w499:T3)
        n156 = Enqueue Element(queue=w501, element=w499, error in (no error)=w503) -> (error out=w502:errorcluster)  [unwired: 1 in, 2 out]
      }
      event "Start": Value Change {
        # "On pressing Start go the start state."
        n157 = event-data() -> ()  [unwired: 1 in, 1 out]
        n158 = Enqueue Element(queue=w506, element=T3 {"Command"=enum."Start", "Data"=variant} ("Car Race Cmd Data Cluster"), error in (no error)=w508) -> (error out=w507:errorcluster)  [unwired: 1 in, 2 out]
      }
      event "Re-Start": Value Change {
        # "Restart the game again."
        n159 = event-data() -> ()  [unwired: 1 in, 3 out]
        n160 = Flush Queue(queue=w514, error in (no error)=w510) -> (queue out=w511:refnum<queue>, error out=w509:errorcluster)  [unwired: 1 out]
        n161 = Enqueue Element(queue=w511, element=T3 {"Command"=enum."Re-Start", "Data"=variant} ("Car Race Cmd Data Cluster"), error in (no error)=w509) -> (error out=w515:errorcluster)  [unwired: 1 in, 2 out]
      }
      event "Stop": Value Change {
        # "Stop the game."
        n162 = event-data() -> ()  [unwired: 1 in, 1 out]
        n163 = Enqueue Element(queue=w518, element=T3 {"Command"=enum."Stop", "Data"=variant} ("Car Race Cmd Data Cluster"), error in (no error)=w520) -> (error out=w519:errorcluster)  [unwired: 1 in, 2 out]
      }
    }
    n164 = Unbundle By Name(w491) -> ("status"=w490:bool)
    n165 = Or(x=w490, y=w493) -> (x .or. y?=w492:bool)
  }
  n166 = Merge Errors(w3, w8) -> (w9:errorcluster)
  n167 = Release Queue(queue=w19, error in (no error)=w9) -> (error out=w7:errorcluster)  [unwired: 1 in, 2 out]
  n168 = call <vilib>:"Simple Error Handler.vi"("error in (no error)"=w7) -> ()  [unwired: 4 in, 5 out]
